vi "GetAllDepsPath.vi"(8 "error in (no error)":errorcluster, 11 "Source Folder Path":path=path "C:/sw-deps-monitor/Source") -> (0 "error out":errorcluster, 3 "All .deps in Repo":path[](array[path]))   [LabVIEW 2019, in "DepsWatch.lvlib"]
uses:
  DepsWatch.lvlib
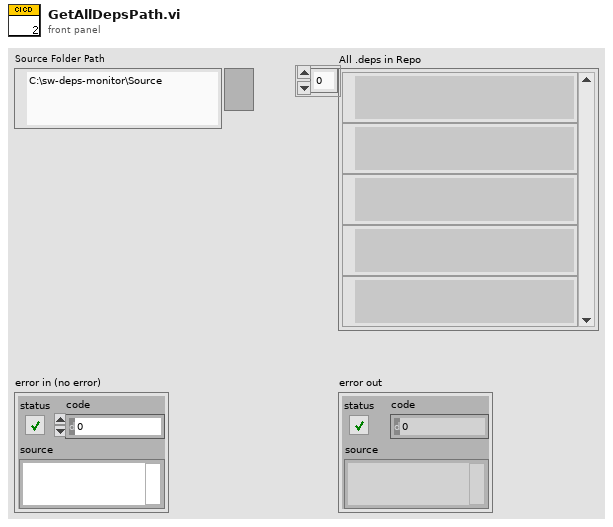
[diagram p1: front panel]
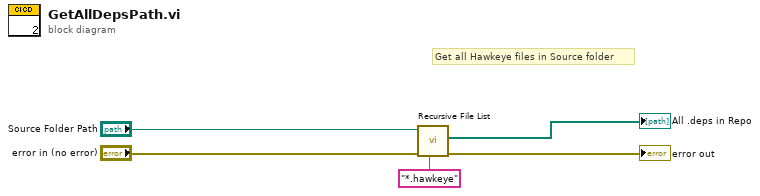
[diagram p0: block diagram]
diagram:
  # "Get all Hawkeye files in Source folder"
  n1 = call <vilib>:"Recursive File List.vi"("pattern"="*.hawkeye", "error in (no error)"="error in (no error)", "Folder Path"="Source Folder Path") -> ("error out"=→"error out":errorcluster, "All Files in Dir"=→"All .deps in Repo":path[])  [unwired: 4 in, 3 out]
